vi "Teleop.vi"(10 "Match Info":T1={"Autonomous Elapsed Seconds"=0.0, "TeleOp Elapsed Seconds"=0.0, "Disabled Elapsed Seconds"=0.0, "Visited Autonomous"=FALSE, "Visited TeleOp"=FALSE, "Visited Disabled"=FALSE, "Autonomous Settings"={"Autonomous Style"=enum."Independent", "VI Refnum"=refnum}}, 11 "Call Context":T2) -> ()   [LabVIEW 2015]
doc: "This VI is called for each TeleOp packet received from the DS where the robot is not disabled. It is often used to read from the joysticks and update I/O or to update setpoints for timed control loops. It should complete and return within 20 milliseconds or it may miss DS packets."
uses:
  <vilib>/Rock Robotics/WPI/DriverStation/WPI_DriverStationDerivedRobotMode.ctl
  <vilib>/Rock Robotics/WPI/DriverStation/WPI_DriverStationMatch Info.ctl
  <vilib>/Rock Robotics/WPI/Utilities/WPI_GetSetVariantRefNum.vi
  <vilib>/Rock Robotics/Network Tables/NT Read Boolean.vi
  <vilib>/Rock Robotics/Network Tables/NT Read Number.vi
  <vilib>/Rock Robotics/Network Tables/NT Write Numeric Array.vi
  <vilib>/Rock Robotics/Network Tables/NT Write Boolean Array.vi
panel:
  out "Reverse Limit Switch Closed":bool
  out "Forward Limit Switch Closed":bool
  out "Sample Slider 0":dbl(slide) scale=0.0..5.0
  out "Sample Boolean 1":bool
  out "Sample Boolean 0":bool
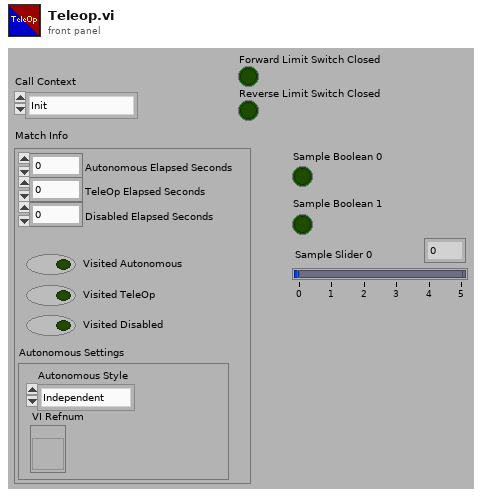
[diagram p1: front panel]
types:
  T1 = typedef "WPI_DriverStationMatch Info.ctl" = cluster{"Autonomous Elapsed Seconds":dbl, "TeleOp Elapsed Seconds":dbl, "Disabled Elapsed Seconds":dbl, "Visited Autonomous":bool, "Visited TeleOp":bool, "Visited Disabled":bool, "Autonomous Settings":cluster{"Autonomous Style":enum16{"Iterative", "Independent"}, "VI Refnum":refnum<vi>}}
  T2 = typedef "WPI_DriverStationDerivedRobotMode.ctl" = enum16{"Init", "Execute", "Stop"}
  T3 = typedef "WPI_RobotDriveDevRef.ctl" = cluster{"DevStatus":errorcluster, "Motors[]":T4[], "Square Inputs":bool, "Max Output":dbl}
  T4 = typedef "WPI_MotorControlDeviceRef.ctl" = cluster{"DeviceStatus":errorcluster, "Type":T5, "PWM":cluster{"PWM Channel":T6, "DeadBand":T7}, "CAN":cluster{"Device Number":u8, "Control Mode":T8, "Semaphore":T9, "Max Vout":dbl, "TalonSRX Control Mode":T10}, "Invert":bool}
  T5 = typedef "WPI_MotorControlType.ctl" = enum16{"PWM", "CAN", "CANTalonSRX"}
  T6 = typedef "FPGA_DIOPWMChannel.ctl" = enum8{"PWM 0", "PWM 1", "PWM 2", "PWM 3", "PWM 4", "PWM 5", "PWM 6", "PWM 7", "PWM 8", "PWM 9", "PWM MXP 0", "PWM MXP 1", "PWM MXP 2", "PWM MXP 3", "PWM MXP 4", "PWM MXP 5", "PWM MXP 6", "PWM MXP 7", "PWM MXP 8", "PWM MXP 9", "Invalid"}
  T7 = typedef "WPI_PWMDeadband.ctl" = cluster{"Name":string, "maxPositivePwm":i32, "minPositivePwm":i32, "centerPwm":i32, "maxNegativePwm":i32, "minNegativePwm":i32, "angularRange":u16}
  T8 = typedef "WPI_CANJaguar_ControlMode.ctl" = enum8{"Percent VBus", "Current", "Speed", "Position", "Voltage"}
  T9 = typedef "Semaphore RefNum" = refnum<k1>
  T10 = typedef "WPI_CANTalonSRX_APIControlMode.ctl" = enum8{"Percent VBus", "Speed", "Position", "Slave", "Unchanged / Invalid", "Voltage Compensation", "Current", "Motion Profile"}
  T11 = typedef "WPI_JoystickDevRef.ctl" = cluster{"Device":T12}
  T12 = typedef "WPI_JoystickDeviceEnum.ctl" = enum16{"USB 0", "USB 1", "USB 2", "USB 3", "USB 4", "USB 5"}
  T13 = typedef "WPI_CANTalonSRX_GlobalStatus.ctl" = cluster{"Applied Throttle":dbl, "Module Enabled":bool, "CAN Error":errorcluster, "Closed Loop Error":dbl, "Forward Limit Switch Closed":bool, "Reverse Limit Switch Closed":bool, "Sensor Position":dbl, "Sensor Velocity":dbl, "Current":dbl, "Sticky Fault - Over Temp":bool, "Sticky Fault - Under Voltage":bool, "Sticky Fault - Forward Limit":bool, "Sticky Fault - Reverse Limit":bool, "Sticky Fault - Forward Soft Limit":bool, "Sticky Fault - Reverse Soft Limit":bool, "Brake is Enabled":bool, "Encoder Position":dbl, "Encoder Velocity":dbl, "Encoder Index Count":dbl, "Encoder A Pin State":bool, "Encoder B Pin State":bool, "Encoder Index Pin State":bool, "Analog In":dbl, "Analog In Velocity":dbl, "Temperature (C)":dbl, "Battery Voltage":dbl, "Control 5 Is Supported":bool, "Current Profile Slot Select":dbl, "Pos Div 8":bool, "Vel Div 4":bool, "Pulse Width Position":i32, "Pulse Width Velocity":i32, "Pulse Width Rise To Rise (us)":i32, "Pulse Width Rise To Fall (us)":i32, "Mot Prof Active Is Under Run":bool, "Mot Prof Active Has Under Run":bool, "Mot Prof Active Is Last":bool, "Mot Prof Active Velocity Only":bool, "Mot Prof Active Is Valid":bool, "Mot Prof Buffer Is Full":bool, "Mot Prof Active Profile Slot Select":i32, "Mot Prof NextID":i32, "Mot Prof Count":i32, "Mot Prof Active Velocity":dbl, "Mot Prof Active Position":dbl, "Mot Prof Output Enable":i32}
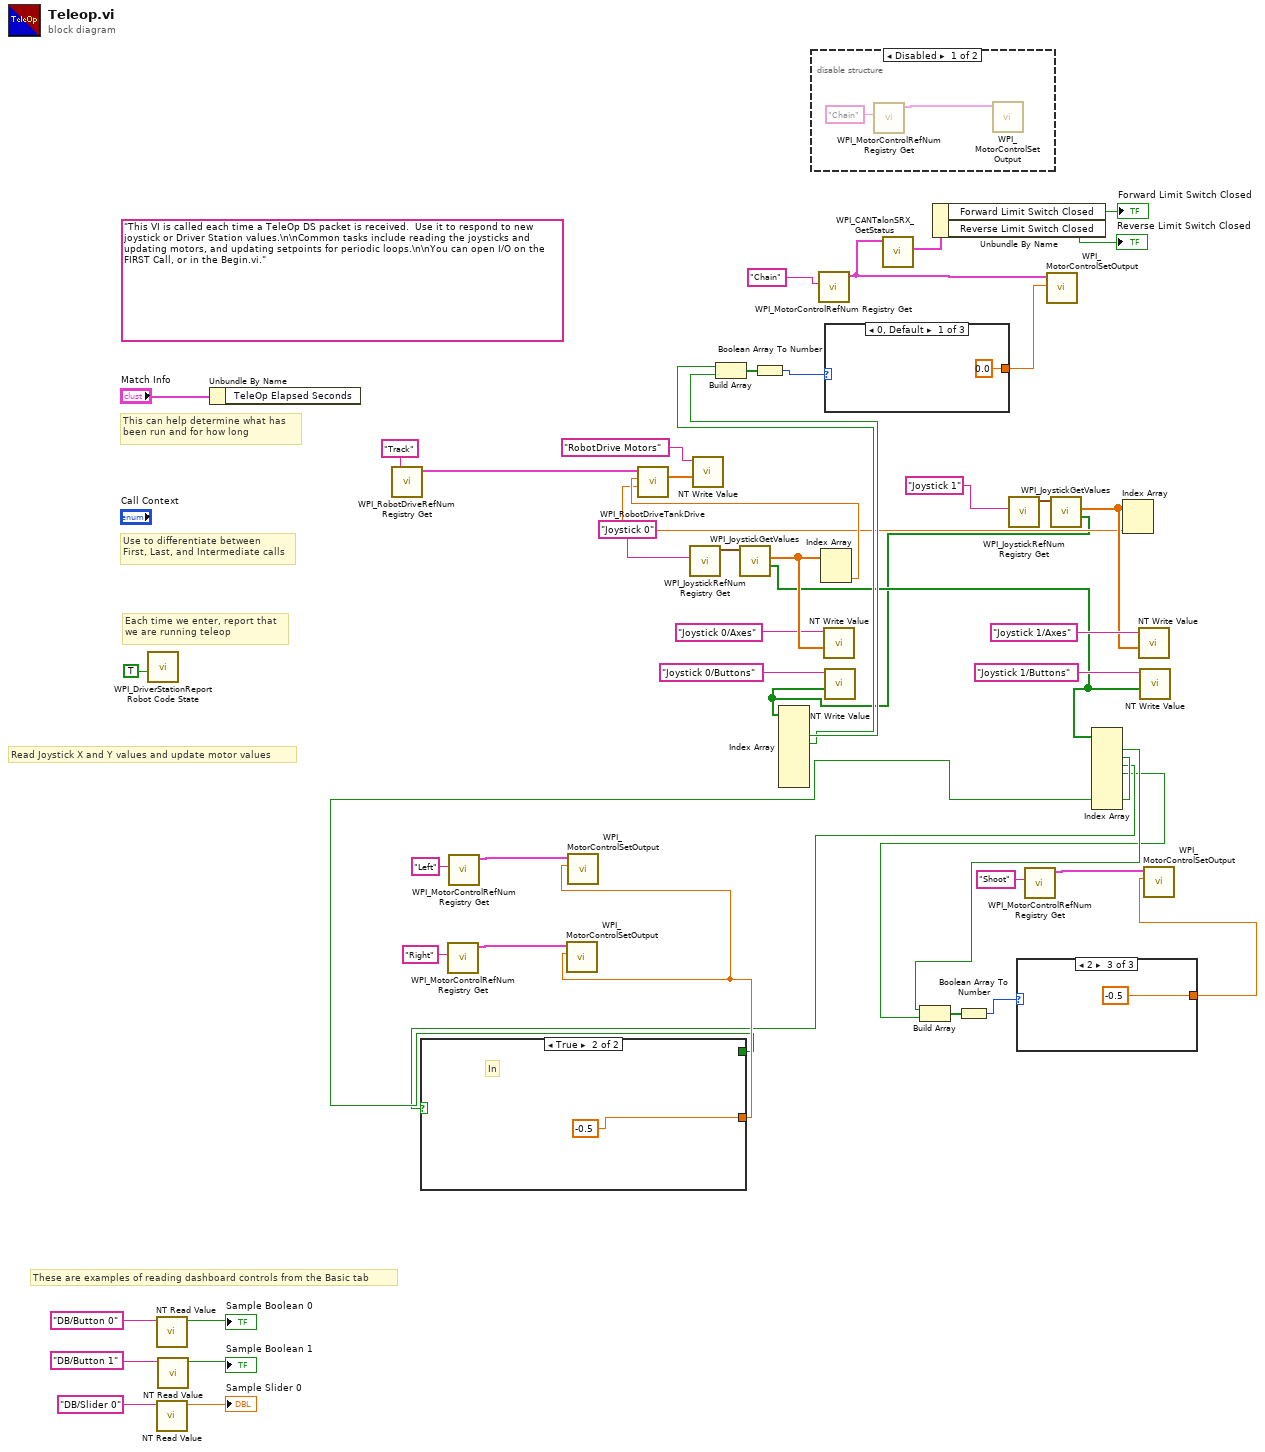
[diagram p0: block diagram]
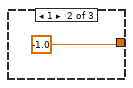
[diagram p2: hidden frame]
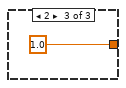
[diagram p3: hidden frame]
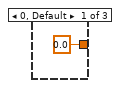
[diagram p5: hidden frame]
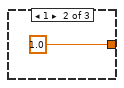
[diagram p6: hidden frame]
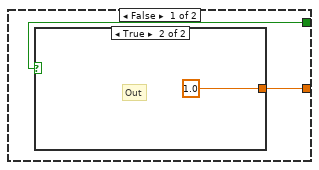
[diagram p7: hidden frame]
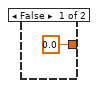
[diagram p8: hidden frame]
diagram:
  (unwired) "This VI is called each time a TeleOp DS packet is received.  Use it to respond to new joystick or Driver Station values.\n\nCommon tasks include reading the joysticks and updating motors, and updating setpoints for periodic loops.\n\nYou can open I/O on the FIRST Call, or in the Begin.vi."
  # "These are examples of reading dashboard controls from the Basic tab"
  # "Each time we enter, report that\nwe are running teleop"
  # "Use to differentiate between\nFirst, Last, and Intermediate calls"
  # "This can help determine what has\nbeen run and for how long"
  # "Read Joystick X and Y values and update motor values"
  n1 = call <vilib>:"WPI_DriverStationReport Robot Code State.vi"("TeleOp"=TRUE ("Autonomous")) -> ()  [unwired: 10 in, 1 out]
  n2 = call-poly <vilib>:"NT Read Value.vi"("Name"="DB/Button 0" ("refnum name")) -> ("Boolean"=→"Sample Boolean 0":bool)  [unwired: 9 in, 1 out]
  n3 = call-poly <vilib>:"NT Read Value.vi"("Name"="DB/Slider 0" ("refnum name")) -> ("Numeric"=→"Sample Slider 0":dbl)  [unwired: 9 in, 1 out]
  n4 = call-poly <vilib>:"NT Read Value.vi"("Name"="DB/Button 1" ("refnum name")) -> ("Boolean"=→"Sample Boolean 1":bool)  [unwired: 9 in, 1 out]
  n5 = Unbundle By Name("Match Info") -> ()  [unwired: 1 out]
  n6 = call <vilib>:"WPI_RobotDriveRefNum Registry Get.vi"("refnum name"="Track") -> ("RobotDriveDevRef"=w48:T3)  [unwired: 1 in, 9 out]
  n7 = call <vilib>:"WPI_MotorControlRefNum Registry Get.vi"("refnum name"="Right") -> ("MotorControlDevRef"=w22:T4)  [unwired: 9 in, 1 out]
  n8 = call <vilib>:"WPI_MotorControlRefNum Registry Get.vi"("refnum name"="Left") -> ("MotorControlDevRef"=w25:T4)  [unwired: 9 in, 1 out]
  n9 = call <vilib>:"WPI_JoystickRefNum Registry Get.vi"("refnum name"="Joystick 0") -> ("JoystickDevRef"=w35:T11)  [unwired: 1 in, 9 out]
  n10 = call <vilib>:"WPI_JoystickGetValues.vi"("JoystickDevRef"=w35) -> ("Buttons"=w2:bool[], "Axes"=w38:dbl[])  [unwired: 6 in, 3 out]
  n11 = disable-structure shown="Disabled" {
    frame Disabled {
      n12 = call <vilib>:"WPI_MotorControlRefNum Registry Get.vi"("refnum name"="Chain") -> ("MotorControlDevRef"=w51:T4)  [unwired: 9 in, 1 out]
      n13 = call <vilib>:"WPI_MotorControlSetOutput.vi"("MotorControlDevRef"=w51) -> ()  [unwired: 8 in, 3 out]
    }
    frame Enabled {
    }
  }
  n14 = call <vilib>:"WPI_MotorControlRefNum Registry Get.vi"("refnum name"="Chain") -> ("MotorControlDevRef"=w14:T4)  [unwired: 9 in, 1 out]
  n15 = Index Array(array=w38) -> (element #2=w4:dbl)  [unwired: 2 in, 1 out]
  n16 = call-poly <vilib>:"NT Write Value.vi"("Numeric Array"=w38, "Name"="Joystick 0/Axes") -> ()  [unwired: 9 in, 1 out]
  n17 = call <vilib>:"WPI_CANTalonSRX_GetStatus.vi"("CAN Talon SRX Ref"=w14) -> ("Talon SRX Status"=w13:T13)  [unwired: 8 in, 2 out]
  n18 = Unbundle By Name(w13) -> ("Forward Limit Switch Closed"=→"Forward Limit Switch Closed":bool, "Reverse Limit Switch Closed"=→"Reverse Limit Switch Closed":bool)
  n19 = call <vilib>:"WPI_JoystickRefNum Registry Get.vi"("refnum name"="Joystick 1") -> ("JoystickDevRef"=w33:T11)  [unwired: 9 in, 1 out]
  n20 = call <vilib>:"WPI_MotorControlRefNum Registry Get.vi"("refnum name"="Shoot") -> ("MotorControlDevRef"=w27:T4)  [unwired: 9 in, 1 out]
  n21 = call <vilib>:"WPI_JoystickGetValues.vi"("JoystickDevRef"=w33) -> ("Buttons"=w1:bool[], "Axes"=w30:dbl[])  [unwired: 6 in, 3 out]
  n22 = Index Array(array=w1) -> (element #2=w6:bool, element #3=w5:bool)  [unwired: 8 in, 6 out]
  n23 = Build Array(w5, w6) -> (w17:bool[])
  n24 = Boolean Array To Number(Boolean array=w17) -> (number=w16:u32)
  n25 = case shown="0, Default" w16 {
    tunnel: [0.0 ("Output") -1.0 ("Output") 1.0 ("Output")] -> w15
    frame 0, Default {
    }
    frame 1 {
    }
    frame 2 {
    }
  }
  n26 = call-poly <vilib>:"NT Write Value.vi"("Boolean Array"=w1, "Name"="Joystick 0/Buttons") -> ()  [unwired: 9 in, 1 out]
  n27 = call <vilib>:"WPI_MotorControlSetOutput.vi"("Output"=w15, "MotorControlDevRef"=w14) -> ()  [unwired: 7 in, 3 out]
  n28 = Index Array(array=w2) -> (element #1=w9:bool, element #2=w20:bool, element #3=w19:bool, element #4=w7:bool)  [unwired: 8 in, 4 out]
  n29 = case shown="True" w19 {
    tunnel: w20 -> [w57 _]
    tunnel: [w56 -0.5 ("X axis value")] -> w21
    frame False {
      n30 = case shown="True" w57 {
        tunnel: [0.0 ("Y axis value") 1.0 ("Y axis value")] -> w56
        frame False {
        }
        frame True {
          # "Out"
        }
      }
    }
    frame True {
      # "In"
    }
  }
  n31 = call <vilib>:"WPI_MotorControlSetOutput.vi"("Output"=w21, "MotorControlDevRef"=w22) -> ()  [unwired: 7 in, 3 out]
  n32 = call <vilib>:"WPI_MotorControlSetOutput.vi"("Output"=w21, "MotorControlDevRef"=w25) -> ()  [unwired: 7 in, 3 out]
  n33 = Build Array(w9, w7) -> (w10:bool[])
  n34 = Boolean Array To Number(Boolean array=w10) -> (number=w8:u32)
  n35 = case shown="2" w8 {
    tunnel: [0.0 ("Motor Output") 1.0 ("Motor Output") -0.5 ("Motor Output")] -> w26
    frame 0, Default {
    }
    frame 1 {
    }
    frame 2 {
    }
  }
  n36 = Index Array(array=w30) -> (element #2=w3:dbl)  [unwired: 2 in, 1 out]
  n37 = call <vilib>:"WPI_RobotDriveTankDrive.vi"("Right axis value"=w3, "Left axis value"=w4, "RobotDriveDevRef"=w48) -> ("Motor Values"=w40:dbl[])  [unwired: 6 in, 2 out]
  n38 = call-poly <vilib>:"NT Write Value.vi"("Numeric Array"=w40, "Name"="RobotDrive Motors") -> ()  [unwired: 9 in, 1 out]
  n39 = call-poly <vilib>:"NT Write Value.vi"("Numeric Array"=w30, "Name"="Joystick 1/Axes") -> ()  [unwired: 9 in, 1 out]
  n40 = call-poly <vilib>:"NT Write Value.vi"("Boolean Array"=w2, "Name"="Joystick 1/Buttons") -> ()  [unwired: 9 in, 1 out]
  n41 = call <vilib>:"WPI_MotorControlSetOutput.vi"("Output"=w26, "MotorControlDevRef"=w27) -> ()  [unwired: 7 in, 3 out]
